vi "Rotation Control.vi"(3 "Filtered Ohmega":dbl, 4 "Original Difference":dbl, 5 "Alpha Desired":dbl, 6 "Alpha In":dbl) -> (0 "Maneuver Complete?":bool, 1 "Counter-ClkWise Rot Ctrl":bool, 2 "Clockwise Rot Ctrl":bool)   [LabVIEW 2012]
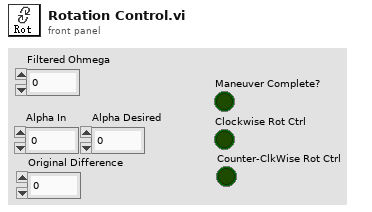
[diagram p1: front panel]
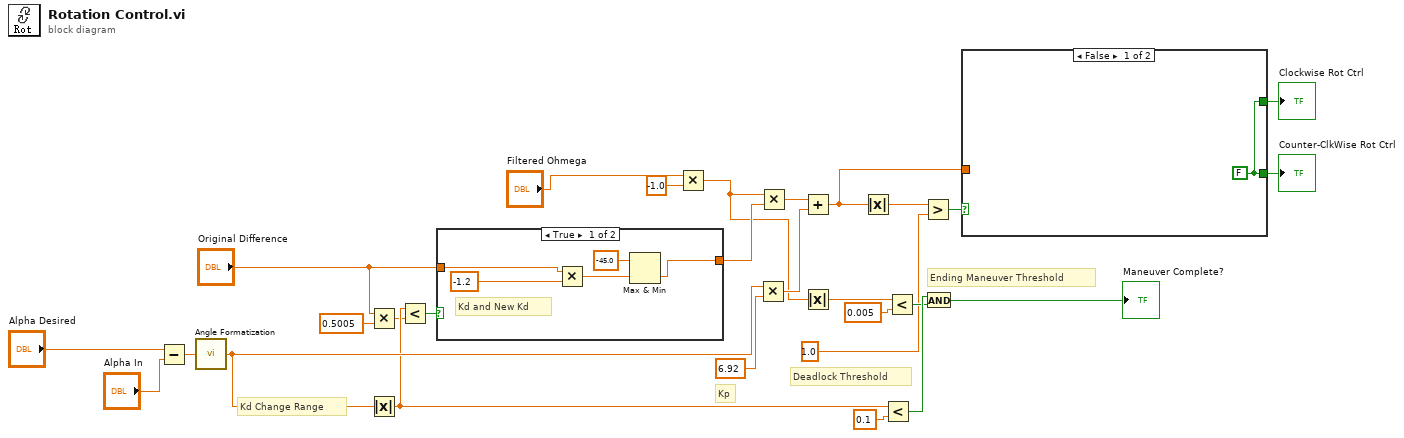
[diagram p0: block diagram]
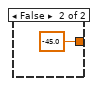
[diagram p2: hidden frame]
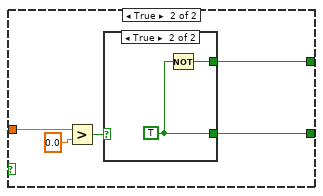
[diagram p3: hidden frame]
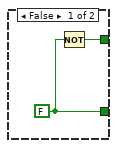
[diagram p4: hidden frame]
diagram:
  # "Deadlock Threshold"
  # "Ending Maneuver Threshold"
  # "Kp"
  # "Kd Change Range"
  n1 = Subtract(x="Alpha Desired", y="Alpha In") -> (x-y=w28:dbl)
  n2 = call "Angle Formatization.vi"("Alpha"=w28) -> ("Alpha Formatized"=w21:dbl)
  n3 = Multiply(x="Original Difference", y=0.5005) -> (x*y=w11:dbl)
  n4 = Absolute Value(x=w21) -> (abs(x)=w13:dbl)
  n5 = Less?(x=w13, y=w11) -> (x < y?=w10:bool)
  n6 = case shown="True" w10 {
    tunnel: [w29 -45.0 ("y")] -> w25
    tunnel: "Original Difference" -> [w32 _]
    frame True {
      # "Kd and New Kd"
      n7 = Multiply(x=w32, y=-1.2) -> (x*y=w31:dbl)
      n8 = Max & Min(x=-45.0 ("y"), y=w31) -> (min(x,y)=w29:dbl)  [unwired: 1 out]
    }
    frame False {
    }
  }
  n9 = Multiply(x="Filtered Ohmega", y=-1.0) -> (x*y=w3:dbl)
  n10 = Multiply(x=w21, y=6.92) -> (x*y=w26:dbl)
  n11 = Multiply(x=w3, y=w25) -> (x*y=w18:dbl)
  n12 = Add(x=w18, y=w26) -> (x+y=w22:dbl)
  n13 = Absolute Value(x=w3) -> (abs(x)=w17:dbl)
  n14 = Absolute Value(x=w22) -> (abs(x)=w24:dbl)
  n15 = Less?(x=w13, y=0.1) -> (x < y?=w19:bool)
  n16 = Less?(x=w17, y=0.005) -> (x < y?=w15:bool)
  n17 = Greater?(x=w24, y=1.0 ("x")) -> (0:w23:bool)
  n18 = And(x=w19, y=w15) -> (x .and. y?=→"Maneuver Complete?":bool)
  n19 = case shown="False" w23 {
    tunnel: [w35 w40] -> w5
    tunnel: [w35 w38] -> w6
    tunnel: w22 -> [_ w37]
    frame False {
      w35 = FALSE
    }
    frame True {
      n20 = Greater?(x=w37, y=0.0) -> (0:w39:bool)
      n21 = case shown="True" w39 {
        tunnel: [w42 w44] -> w40
        tunnel: [w41 w43] -> w38
        frame False {
          w42 = FALSE ("clkwis")
          n22 = Not(x=w42) -> (.not. x?=w41:bool)
        }
        frame True {
          w44 = TRUE ("clkwis")
          n23 = Not(x=w44) -> (.not. x?=w43:bool)
        }
      }
    }
  }
  "Clockwise Rot Ctrl" <- w6
  "Counter-ClkWise Rot Ctrl" <- w5
